vi "Main2.vi"() -> ()   [LabVIEW 2018]
uses:
  Digit--control.ctl
  multiplier--control.ctl
  tolerance--control.ctl
  temp coeficient--control.ctl
  states--control.ctl
  data--control.ctl
  E-Series Reader/series data--control.ctl
  E-Series Reader/E-Series Reader.lvlib
panel:
  in  "ini filenames":string="e-series files names.ini"
  out "Tem color":u32(colorbox) caption="TC"
  out "3D color":u32(colorbox) caption="3D"
  out "Tol color":u32(colorbox) caption="Tol"
  out "M color":u32(colorbox) caption="M"
  out "2D color":u32(colorbox) caption="2D"
  out "1D color":u32(colorbox) caption="1D"
  in  "Temp Coef":T1
  in  "3° Digit":T2
  in  "Band number":u8=4 min=4 max=6 step=1
  out "Omhs":dbl format="%#_3p"
  out "in E12?":bool caption="In E12 Series?"
  out "in E24?":bool caption="In E24 Series?"
  in  "Tolerance":T3=enum."Gold - 5%"
  in  "Multiplier":T4
  in  "2° Digit":T2
  in  "1° Digit":T2
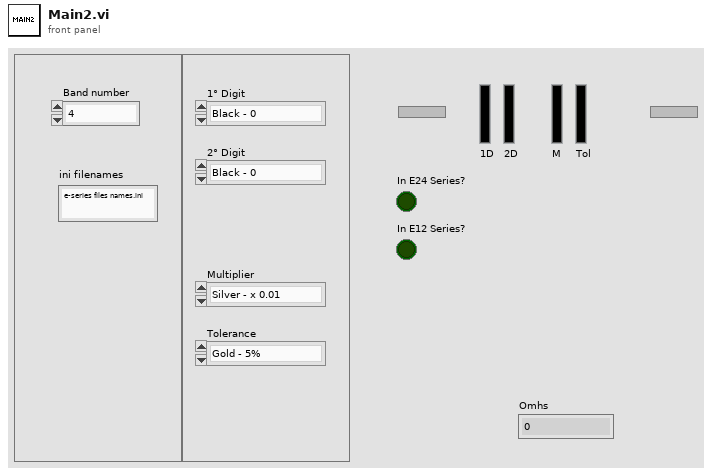
[diagram p1: front panel]
types:
  T1 = typedef "temp coeficient--control.ctl" = enum16{"Grey - 1 ppm/K", "Violet - 5 ppm/K", "Blue - 10 ppm/K", "Green - 20 ppm/K", "Yellow - 25 ppm/K", "Orange - 15 ppm/K", "Red - 50 ppm/K", "Brown - 100 ppm/K", "Black - 250 ppm/K"}
  T2 = typedef "Digit--control.ctl" = enum16{"Black - 0", "Brown - 1", "Red - 2", "Orange - 3", "Yellow - 4", "Green - 5", "Blue - 6", "Violet - 7", "Grey - 8", "White - 9"}
  T3 = typedef "tolerance--control.ctl" = enum16{"Gray - 0.05%", "Violet - 0.1%", "Blue - 0.25%", "Green - 0.5%", "Brown - 1%", "Red - 2%", "Gold - 5%", "Silver - 10%", "None - 20%"}
  T4 = typedef "Multiplier--control.ctl" = enum16{"Silver - x 0.01", "Gold - x 0.1 ", "Black - x 1", "Brown - x 10", "Red - x 100", "Orange - x 1k", "Yellow - x 10k", "Green - 100k", "Blue - x 1M", "Violet - x10 M", "Grey - x 100M", "White - x 1G"}
  T5 = typedef "data--control.ctl" = cluster{"1d Refn":refnum<vi>, "2d Refn":refnum<vi>, "3d Ref":refnum<vi>, "Mult Refn":refnum<vi>, "Tol Refn":refnum<vi>, "Band Number":u8, "Series Data":T6, "In E24?":bool, "In E12?":bool, "1D sel":T2, "2D sel":T2, "3D sel":T2, "M sel":T7, "Tol sel":T3, "Tem sel":T1, "D1 color":u32, "D2 color":u32, "D3 color":u32, "M color":u32, "Tol color":u32, "Tem color":u32}
  T6 = typedef "E-Series Reader.lvlib/series data--control.ctl" = cluster{"E3":u16[], "E6":u16[], "E12":u16[], "E24":u16[], "E48":u16[], "E96":u16[], "E192":u16[]}
  T7 = typedef "multiplier--control.ctl" = enum16{"Silver - x 0.01", "Gold - x 0.1 ", "Black - x 1", "Brown - x 10", "Red - x 100", "Orange - x 1k", "Yellow - x 10k", "Green - 100k", "Blue - x 1M", "Violet - x10 M", "Grey - x 100M", "White - x 1G"}
  T8 = typedef "states--control.ctl" = enum16{"Initialize", "Hide Inactive Bands", "Read CSV Series", "Set Colors", "Read Parameters", "Set Resistance Colors", "Verify E12 Series", "Verify E24 Series ", "Get Value", "Error", "Shutdown"}
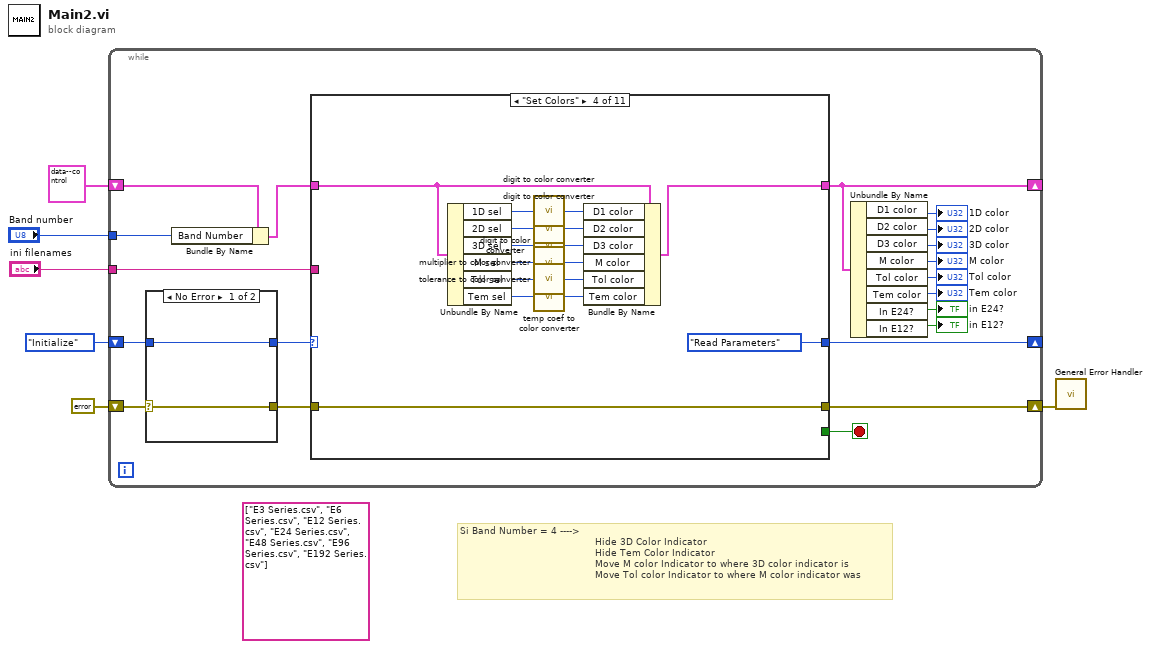
[diagram p0: block diagram]
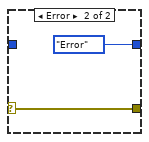
[diagram p2: hidden frame]
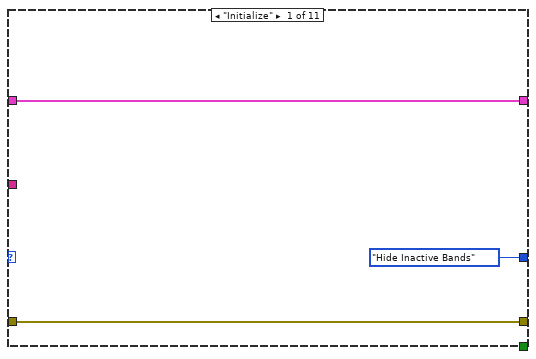
[diagram p3: hidden frame]
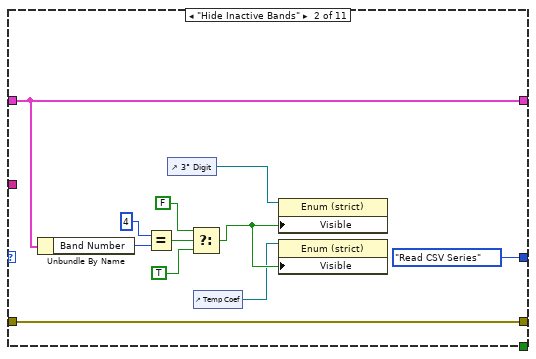
[diagram p4: hidden frame]
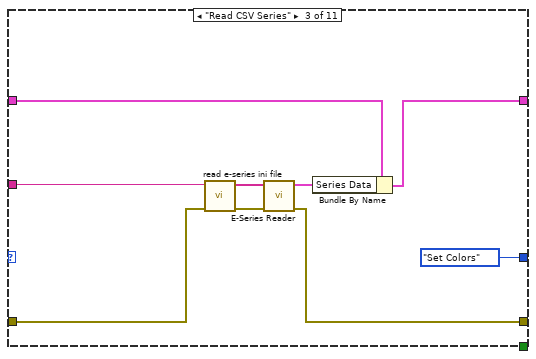
[diagram p5: hidden frame]
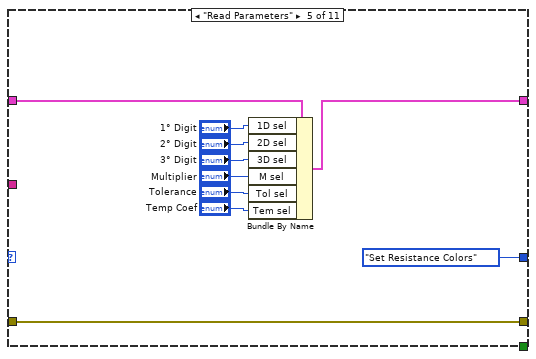
[diagram p6: hidden frame]
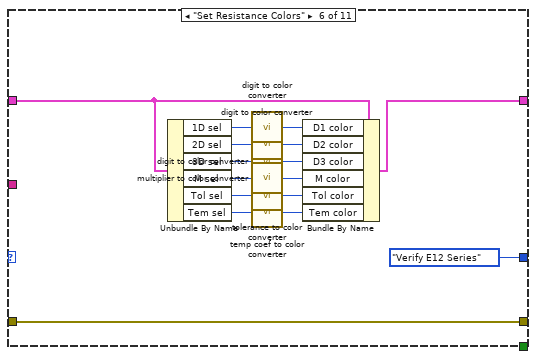
[diagram p7: hidden frame]
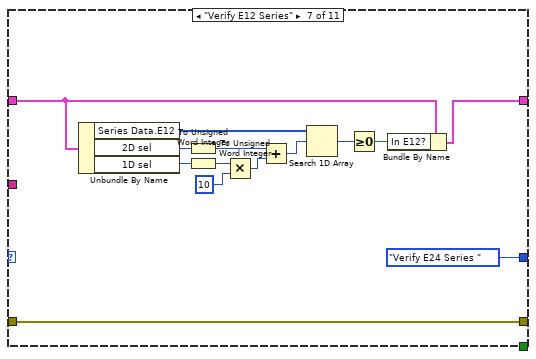
[diagram p8: hidden frame]
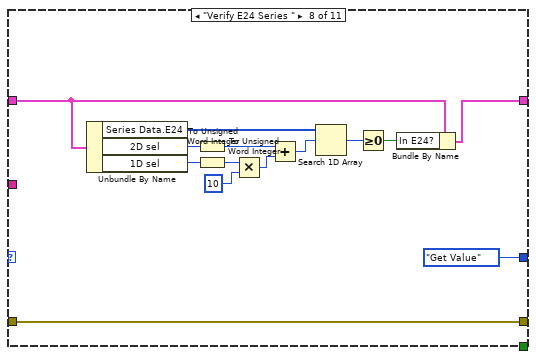
[diagram p9: hidden frame]
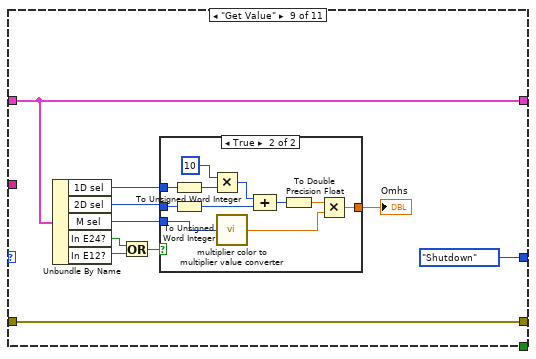
[diagram p10: hidden frame]
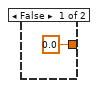
[diagram p11: hidden frame]
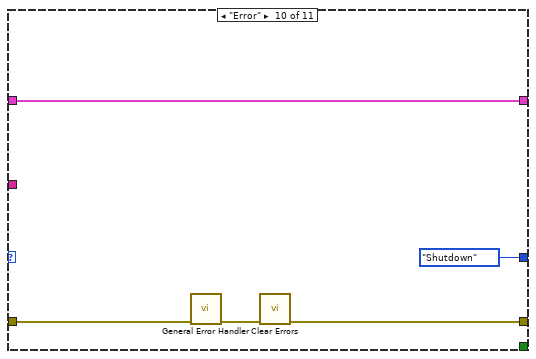
[diagram p12: hidden frame]
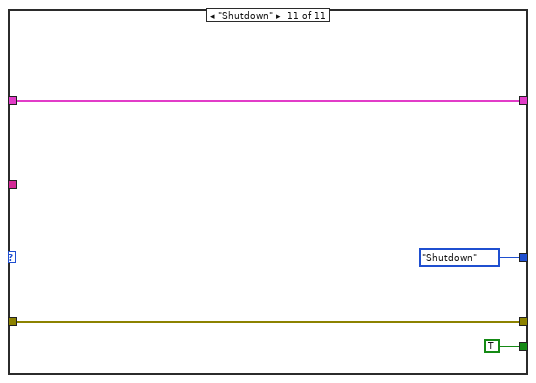
[diagram p13: hidden frame]
diagram:
  (unwired) string[] ["E3 Series.csv", "E6 Series.csv", "E12 Series.csv", "E24 Series.csv", "E48 Series.csv", "E96 Series.csv", "E192 Series.csv"] ("E Series File Names")
  # "Si Band Number = 4 ----> \n                                             Hide 3D Color Indicator\n                                             Hide Tem Color Indicator\n                                             Move M color Indicator to where 3D color indicator is\n                                             Move Tol color Indicator to where M color indicator was"
  n1 = while {
    shift-right: [w21] -> _
    shift-left: states--control."Initialize" -> [w26]
    shift-right: [w22] -> w3
    shift-left: errorcluster {"status"=FALSE, "code"=0, "source"=""} ("error constant") -> [w25]
    shift-right: [w19] -> _
    shift-left: T5 {"1d Refn"=refnum, "2d Refn"=refnum, "3d Ref"=refnum, "Mult Refn"=refnum, "Tol Refn"=refnum, "Band Number"=0, "Series Data"={"E3"=[], "E6"=[], "E12"=[], "E24"=[], "E48"=[], "E96"=[], "E192"=[]}, "In E24?"=FALSE, "In E12?"=FALSE, "1D sel"=enum."Black - 0", "2D sel"=enum."Black - 0", "3D sel"=enum."Black - 0", "M sel"=enum."Silver - x 0.01", "Tol sel"=enum."Gray - 0.05%", "Tem sel"=enum."Grey - 1 ppm/K", "D1 color"=0, "D2 color"=0, "D3 color"=0, "M color"=0, "Tol color"=0, "Tem color"=0} -> [w10]
    tunnel: "Band number" -> [w8]
    tunnel: "ini filenames" -> [w7]
    stop <- w20 stop-if-true
    n2 = case shown="No Error" w25 {
      selector: w25 -> [w27 w30]
      tunnel: w26 -> [w28 _]
      tunnel: [w28 states--control."Error"] -> w24
      tunnel: [w27 w30] -> w23
      frame No Error {
      }
      frame Error {
      }
    }
    n3 = Bundle By Name(cluster=w10, "Band Number"=w8) -> (w9:T5)
    n4 = case shown="\"Set Colors\"" w24 {
      tunnel: w23 -> [w33 w44 w46 w69 w79 w93 w109 w123 w133 w147 w154]
      tunnel: [w33 w44 w51 w69 w79 w93 w109 w123 w133 w148 w154] -> w22
      tunnel: w9 -> [w31 w42 w53 w60 w78 w91 w97 w111 w131 w150 w153]
      tunnel: [w31 w42 w52 w66 w77 w90 w96 w110 w131 w150 w153] -> w19
      tunnel: [states--control."Hide Inactive Bands" states--control."Read CSV Series" states--control."Set Colors" states--control."Read Parameters" states--control."Set Resistance Colors" states--control."Verify E12 Series" states--control."Verify E24 Series " states--control."Get Value" states--control."Shutdown" states--control."Shutdown" states--control."Shutdown"] -> w21
      tunnel: [_ _ _ _ _ _ _ _ _ _ TRUE] -> w20
      tunnel: w7 -> [_ _ w45 _ _ _ _ _ _ _ _]
      frame "Initialize" {
      }
      frame "Hide Inactive Bands" {
        n5 = Unbundle By Name(w42) -> ("Band Number"=w41:u8)
        n6 = Equal?(x=u8 4, y=w41) -> (x = y?=w39:bool)
        n7 = control-ref of="3° Digit"() -> (w35:refnum<vi>)
        n8 = Select(t=FALSE, s=w39, f=TRUE) -> (s? t:f=w36:bool)
        n9 = control-ref of="Temp Coef"() -> (w34:refnum<vi>)
        n10 = property class="Enum (strict)"(reference=w35, "Visible"=w36) -> ()  [unwired: 1 in, 2 out]
        n11 = property class="Enum (strict)"(reference=w34, "Visible"=w36) -> ()  [unwired: 1 in, 2 out]
      }
      frame "Read CSV Series" {
        n12 = call "read e-series ini file.vi"("error in (no error)"=w46, "ini filename"=w45) -> ("error out"=w47:errorcluster, "File Names"=w48:string[])  [unwired: 8 in]
        n13 = call "E-Series Reader.vi"("error in"=w47, "E Series File Names"=w48) -> ("error out"=w51:errorcluster, "Series Data"=w50:T6)  [unwired: 8 in]
        n14 = Bundle By Name(cluster=w53, "Series Data"=w50) -> (w52:T5)
      }
      frame "Set Colors" {
        n15 = Unbundle By Name(w60) -> ("1D sel"=w59:T2, "2D sel"=w58:T2, "3D sel"=w57:T2, "M sel"=w56:T7, "Tol sel"=w55:T3, "Tem sel"=w54:T1)
        n16 = call "digit to color converter.vi"("Digit select"=w59) -> ("Digit color"=w68:u32)  [unwired: 4 in]
        n17 = call "digit to color converter.vi"("Digit select"=w58) -> ("Digit color"=w67:u32)  [unwired: 4 in]
        n18 = call "digit to color converter.vi"("Digit select"=w57) -> ("Digit color"=w64:u32)  [unwired: 4 in]
        n19 = call "multiplier to color converter.vi"("Multiplier select"=w56) -> ("Multiplier color"=w63:u32)  [unwired: 6 in]
        n20 = call "tolerance to color converter.vi"("Tolerance select"=w55) -> ("Tolerance Color"=w62:u32)  [unwired: 6 in]
        n21 = call "temp coef to color converter.vi"("Temp Coef select"=w54) -> ("Temp Coef Color"=w61:u32)  [unwired: 6 in]
        n22 = Bundle By Name(cluster=w60, "D1 color"=w68, "D2 color"=w67, "D3 color"=w64, "M color"=w63, "Tol color"=w62, "Tem color"=w61) -> (w66:T5)
      }
      frame "Read Parameters" {
        n23 = Bundle By Name(cluster=w78, "1D sel"="1° Digit", "2D sel"="2° Digit", "3D sel"="3° Digit", "M sel"="Multiplier", "Tol sel"="Tolerance", "Tem sel"="Temp Coef") -> (w77:T5)
      }
      frame "Set Resistance Colors" {
        n24 = Unbundle By Name(w91) -> ("1D sel"=w94:T2, "2D sel"=w92:T2, "3D sel"=w83:T2, "M sel"=w87:T7, "Tol sel"=w86:T3, "Tem sel"=w81:T1)
        n25 = call "digit to color converter.vi"("Digit select"=w94) -> ("Digit color"=w89:u32)  [unwired: 4 in]
        n26 = call "digit to color converter.vi"("Digit select"=w92) -> ("Digit color"=w88:u32)  [unwired: 4 in]
        n27 = call "digit to color converter.vi"("Digit select"=w83) -> ("Digit color"=w82:u32)  [unwired: 4 in]
        n28 = call "multiplier to color converter.vi"("Multiplier select"=w87) -> ("Multiplier color"=w84:u32)  [unwired: 6 in]
        n29 = call "tolerance to color converter.vi"("Tolerance select"=w86) -> ("Tolerance Color"=w85:u32)  [unwired: 6 in]
        n30 = call "temp coef to color converter.vi"("Temp Coef select"=w81) -> ("Temp Coef Color"=w80:u32)  [unwired: 6 in]
        n31 = Bundle By Name(cluster=w91, "D1 color"=w89, "D2 color"=w88, "D3 color"=w82, "M color"=w84, "Tol color"=w85, "Tem color"=w80) -> (w90:T5)
      }
      frame "Verify E12 Series" {
        n32 = Unbundle By Name(w97) -> ("Series Data.E12"=w101:u16[], "2D sel"=w107:T2, "1D sel"=w106:T2)
        n33 = To Unsigned Word Integer(number=w107) -> (unsigned 16bit integer=w103:u16)
        n34 = To Unsigned Word Integer(number=w106) -> (unsigned 16bit integer=w105:u16)
        n35 = Multiply(x=w105, y=u16 10) -> (x*y=w102:u16)
        n36 = Add(x=w103, y=w102) -> (x+y=w100:u16)
        n37 = Search 1D Array(1D array=w101, element=w100) -> (index of element=w99:i32)  [unwired: 1 in]
        n38 = Greater Or Equal To 0?(x=w99) -> (x >= 0?=w98:bool)
        n39 = Bundle By Name(cluster=w97, "In E12?"=w98) -> (w96:T5)
      }
      frame "Verify E24 Series " {
        n40 = Unbundle By Name(w111) -> ("Series Data.E24"=w115:u16[], "2D sel"=w121:T2, "1D sel"=w120:T2)
        n41 = To Unsigned Word Integer(number=w121) -> (unsigned 16bit integer=w117:u16)
        n42 = To Unsigned Word Integer(number=w120) -> (unsigned 16bit integer=w119:u16)
        n43 = Multiply(x=w119, y=u16 10) -> (x*y=w116:u16)
        n44 = Add(x=w117, y=w116) -> (x+y=w114:u16)
        n45 = Search 1D Array(1D array=w115, element=w114) -> (index of element=w113:i32)  [unwired: 1 in]
        n46 = Greater Or Equal To 0?(x=w113) -> (x >= 0?=w112:bool)
        n47 = Bundle By Name(cluster=w111, "In E24?"=w112) -> (w110:T5)
      }
      frame "Get Value" {
        n48 = Unbundle By Name(w131) -> ("1D sel"=w127:T2, "2D sel"=w126:T2, "M sel"=w125:T7, "In E24?"=w130:bool, "In E12?"=w129:bool)
        n49 = Or(x=w130, y=w129) -> (x .or. y?=w128:bool)
        n50 = case shown="True" w128 {
          tunnel: w127 -> [_ w145]
          tunnel: w126 -> [_ w144]
          tunnel: w125 -> [_ w137]
          tunnel: [0.0 w138] -> w124
          frame False {
          }
          frame True {
            n51 = To Unsigned Word Integer(number=w145) -> (unsigned 16bit integer=w143:u16)
            n52 = To Unsigned Word Integer(number=w144) -> (unsigned 16bit integer=w140:u16)
            n53 = Multiply(x=u16 10 ("y"), y=w143) -> (x*y=w142:u16)
            n54 = call "multiplier color to multiplier value converter.vi"("mult color"=w137) -> ("multiplier"=w136:dbl)  [unwired: 6 in]
            n55 = Compound Arithmetic op=ADD(w142, w140) -> (w139:u16)
            n56 = To Double Precision Float(number=w139) -> (double precision float=w135:dbl)
            n57 = Multiply(x=w135, y=w136) -> (x*y=w138:dbl)
          }
        }
        "Omhs" <- w124
      }
      frame "Error" {
        n58 = call <vilib>:"General Error Handler.vi"("error in (no error)"=w147) -> ("error out"=w146:errorcluster)  [unwired: 10 in, 4 out]
        n59 = call <vilib>:"Clear Errors.vi"("error in (no error)"=w146) -> ("error out"=w148:errorcluster)  [unwired: 5 in, 1 out]
      }
      frame "Shutdown" {
      }
    }
    n60 = Unbundle By Name(w19) -> ("D1 color"=→"1D color":u32, "D2 color"=→"2D color":u32, "D3 color"=→"3D color":u32, "M color"=→"M color":u32, "Tol color"=→"Tol color":u32, "Tem color"=→"Tem color":u32, "In E24?"=→"in E24?":bool, "In E12?"=→"in E12?":bool)
  }
  n61 = call <vilib>:"General Error Handler.vi"("error in (no error)"=w3) -> ()  [unwired: 10 in, 5 out]
